vi "sendValue.vi"(8 "error in (no error)":errorcluster, 10 "data":variant, 11 "azimuthMovingDirection in":refnum<class "azimuthMovingDirection.lvclass">) -> (0 "error out":errorcluster, 2 "function return":i32, 3 "azimuthMovingDirection out":refnum<class "azimuthMovingDirection.lvclass">)   [LabVIEW 2016, in "SALLV_AtDome_Messaging.lvlib" / "azimuthMovingDirection.lvclass"]
uses:
  azimuthMovingDirection.lvclass
  ts_sallv_AtDome/DataTypes/logevent_azimuthMovingDirection.ctl
  ts_sallv_AtDome/SALLV_AtDome.lvlib
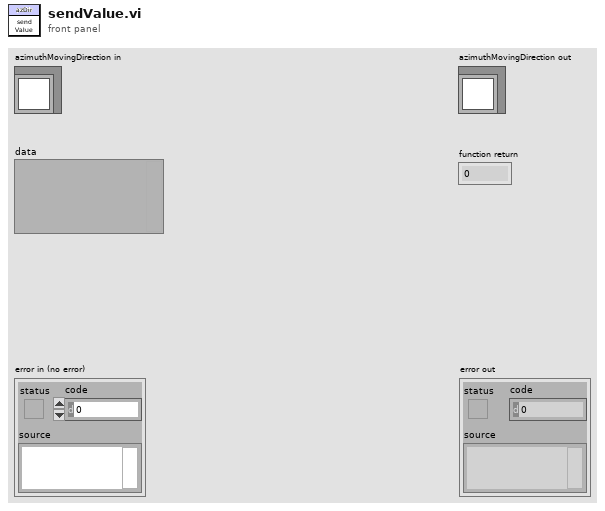
[diagram p1: front panel]
types:
  T1 = typedef "SALLV_AtDome.lvlib/logevent_azimuthMovingDirection.ctl" = cluster{"motionStatus":i32, "priority":i32}
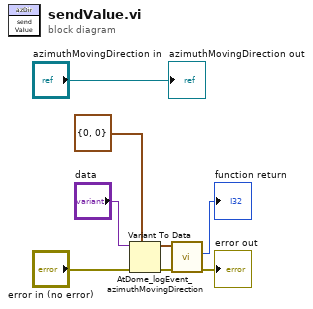
[diagram p0: block diagram]
diagram:
  n1 = Variant To Data(error in="error in (no error)", type=T1 {"motionStatus"=0, "priority"=0} ("logevent_azimuthMovingDirection_Ctl"), Variant="data") -> (data=w4:T1, error out=w5:errorcluster)
  n2 = call "AtDome_logEvent_azimuthMovingDirection.vi"("error in (no error)"=w5, "logevent_azimuthMovingDirection_Ctl"=w4) -> ("error out"=→"error out":errorcluster, "function return"=→"function return":i32)  [unwired: 7 in, 1 out]
  "azimuthMovingDirection out" <- "azimuthMovingDirection in"
